vi "数组转换为矩阵.vi"() -> ()   [LabVIEW 2018]
uses:
  <vilib>/Analysis/Matrix/Datatypes/RealMatrix.ctl
  <vilib>/Analysis/Matrix/Numeric/Conversions/Array To Matrix - RA2.vi
  <vilib>/Analysis/Matrix/NI_Matrix.lvlib
panel:
  in  "停止":bool
  out "Real Matrix":T1 caption="实数矩阵"
  in  "数组":dbl[][](array[numeric])
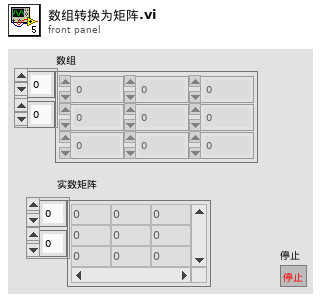
[diagram p1: front panel]
types:
  T1 = typedef "NI_Matrix.lvlib/RealMatrix.ctl" = dbl[][]
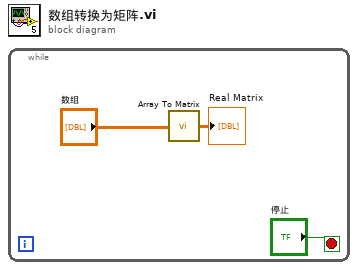
[diagram p0: block diagram]
diagram:
  n1 = while {
    stop <- "停止" stop-if-true
    n2 = call-poly <vilib>:"Array To Matrix.vi"("Real 2D Array"="数组") -> ("Real Matrix"=→"Real Matrix":T1)
  }
